vi "4-Wire Protocol.vi"() -> ()   [LabVIEW 2012]
uses:
  <vilib>/Platform/TimedLoop/XDataNode/timing_clust.ctl
  <vilib>/Platform/TimedLoop/XDataNode/nitl_modes.ctl
  <vilib>/Platform/TimedLoop/XDataNode/wakeup.ctl
  <vilib>/rvi/Analysis/measure/FFT/simModelSupport/niFPGA FFT Sim Properties.ctl
  <vilib>/rvi/Analysis/measure/FFT/simModelSupport/niFPGA FFT Sim Types.ctl
  <vilib>/rvi/Analysis/measure/FFT/simModelSupport/niFpgaFFTSimArithmeticProperties.ctl
  <vilib>/rvi/Analysis/measure/FFT/simModelSupport/niFpgaFFTSimDfxp.ctl
  <vilib>/fxp/LVFixedPointQuantizationPolicyTypeDef.ctl
  <vilib>/rvi/Emulation/niFpgaSctlEmulationRegisterWithScheduler.vi
  <vilib>/rvi/Analysis/common/codeGenErrors/XNode/niFpgaXNodeCodeGenErrorHandle.vi
  <vilib>/rvi/Analysis/measure/FFT/simModelSupport/niFpgaFFTSimModelCore.vi
  <vilib>/rvi/Emulation/niFpgaSctlEmulationScheduler.vi
  <vilib>/Platform/TimedLoop/XDataNode/XDataNode.xnode
  <vilib>/rvi/Analysis/measure/window/XNode/niFPGA Scaled Window.xnode
  <vilib>/rvi/FXPMathLib/basic elements/FxpDiscreteDelay/XNode/nifxpmath_DiscreteDelay.xnode
  <vilib>/rvi/FXPMathLib/FxpMul/XNode/nifxpmath_Multiplier.xnode
  <vilib>/rvi/Analysis/measure/FFT/XNode/niFpgaFFT.xnode
  <vilib>/Platform/TimedLoop/XDataNode/XDNodeRunTimeDep.lvlib
  <vilib>/rvi/FXPMathLib/sim/FxpSim.dll
panel:
  out "Valid Sample Count":u32
  out "SCTL Cycle Count":u32
  out "Data":fxp<+/-,25,24> format="%#.6g"
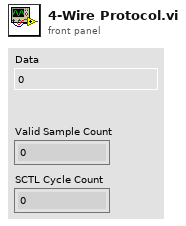
[diagram p1: front panel]
types:
  T1 = typedef "XDNodeRunTimeDep.lvlib/timing_clust.ctl" = cluster{"Expected End [f-1]":u64, "Actual End [f-1]":u64, "Finished Late? [f-1]":bool, "Expected End [i-1]":u64, "Actual End [i-1]":u64, "Finished Late? [i-1]":bool, "Expected Start [i]":u64, "Actual Start [i]":u64, "Expected Start [f]":u64, "Actual Start [f]":u64, "Source Name":string, "Structure Name":string, "Period":i64, "Deadline":i64, "Offset":i64, "Start":i64, "Priority":i32, "Timeout":i32, "Mode":T2, "Wakeup Reason":T3, "Error":errorcluster, "Source Type":string, "Secondary Source Type":string, "Global End Time":u64, "Global Start Time":u64, "Frame Duration":u64, "Iteration Duration":u64, "Assigned CPU":i32, "I/O Scan Engine Mode":u32}
  T2 = typedef "XDNodeRunTimeDep.lvlib/nitl_modes.ctl" = enum32{"No Change", "Process missed periods, maintain original phase", "Discard missed periods, maintain original phase", "Process missed periods, ignore original phase", "Discard missed periods, ignore original phase"}
  T3 = typedef "XDNodeRunTimeDep.lvlib/wakeup.ctl" = enum32{"Normal", "Aborted", "Asynchronous wakeup", "Timing source error", "Timed loop error", "Timeout"}
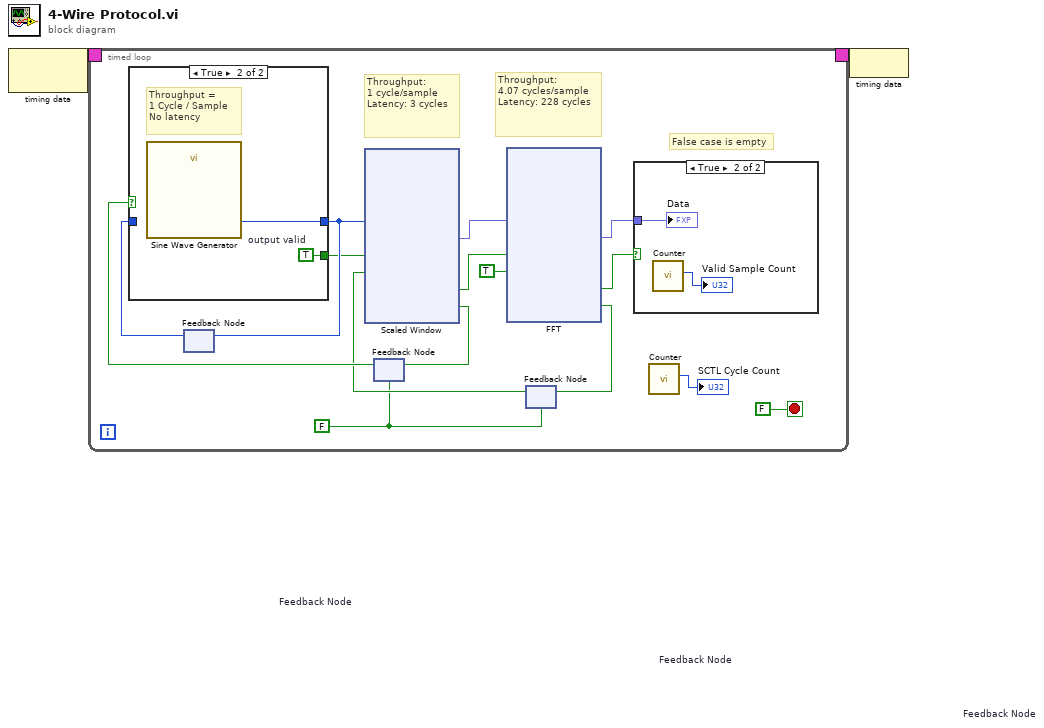
[diagram p0: block diagram]
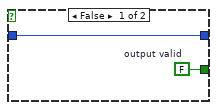
[diagram p3: hidden frame]
diagram:
  n1 = node-c288() -> (w2:T1)  [unwired: 1 in]
  n2 = timed-loop {
    timing: w2 -> [_]
    timing-out: [_] -> w1
    stop <- FALSE stop-if-true
    w3 = FALSE ("ready for input")
    # "False case is empty"
    # "Throughput:\n4.07 cycles/sample\nLatency: 228 cycles"
    # "Throughput:\n1 cycle/sample\nLatency: 3 cycles"
    n3 = feedback #1 "Feedback Node"() -> (w14:i16)  [unwired: 1 in]
    n4 = feedback #2 "Feedback Node"(w3) -> (w16:bool)
    n5 = case shown="True" w16 {
      tunnel: [w47 w49] -> w15
      tunnel: w14 -> [w47 _]
      tunnel: [w46 w48] -> w12
      frame False {
        w46 = FALSE  # output valid
      }
      frame True {
        w48 = TRUE  # output valid
        # "Throughput =\n1 Cycle / Sample\nNo latency"
        n6 = call "Sine Wave Generator"() -> ("sine out"=w49:i16)  [unwired: 15 in]
      }
    }
    n7 = feedback-in #1(w15) -> ()
    n8 = feedback #3 "Feedback Node"(w3) -> (w10:bool)
    n9 = xnode ("Scaled Window")("real data in"=w15, "input valid"=w12, "ready for output"=w10) -> ("real data out"=w13:fxp<+/-,18,17>, "output valid"=w9:bool, "ready for input"=w17:bool)  [unwired: 1 in, 2 out]
    n10 = feedback-in #2(w17) -> ()
    n11 = xnode ("FFT")("real data in"=w13, "input valid"=w9, "ready for output"=TRUE) -> ("real data out"=w7:fxp<+/-,25,24>, "output valid"=w5:bool, "ready for input"=w11:bool)  [unwired: 2 in, 2 out]
    n12 = feedback-in #3(w11) -> ()
    n13 = case shown="True" w5 {
      tunnel: w7 -> [_ w19]
      frame False {
      }
      frame True {
        n14 = call "Counter.vi"() -> ("Count"=→"Valid Sample Count":u32)  [unwired: 10 in]
        "Data" <- w19
      }
    }
    n15 = call "Counter.vi"() -> ("Count"=→"SCTL Cycle Count":u32)  [unwired: 10 in]
  }
  n16 = node-c288(w1) -> ()
